vi "Main Editor UI.vi"() -> ()   [LabVIEW 2014, in "Missing Plugin editor node.lvclass"]
doc: "This is the main view for configuration the behavior of a module in the DCAF standard editor."
uses:
  Missing Plugin editor node.lvclass
  <vilib>/NI/Configuration Framework/Node/NodeRef.ctl
  <vilib>/NI/Configuration Framework/Node/NISE_CEF_Node.lvclass
  <vilib>/NI/AMC/Message Queue.ctl
  <vilib>/NI/AMC/Message.ctl
  <vilib>/NI/Tools/Keyed Array/KeyedArray.ctl
  <vilib>/NI/Configuration Framework/Node/UserEventRef.ctl
  <vilib>/NI/Configuration Framework/Controls/EventCluster.ctl
  <vilib>/NI/Configuration Framework/Node/StopEvent.ctl
  <vilib>/NI/Configuration Framework/Node/RefreshUIEvent.ctl
  <vilib>/NI/Configuration Framework/Node/CacheState.ctl
  <vilib>/NI/Configuration Framework/Node/NodeChangeEvent.ctl
  <vilib>/NI/DCAF/Tag Editor Core/Table API/Available Tag Menu/channel action event.ctl
  <vilib>/NI/DCAF/Tag Editor Core/Table API/Available Tag Menu/dialog output action.ctl
  <vilib>/NI/Tag Bus Module Framework/channel/TBM channel.lvclass
  <vilib>/NI/Tag Bus/tag/tag descriptor.lvclass
  <vilib>/NI/DCAF/Tag Editor Core/Table API/Table Manager/Call Back Ref Type Def.ctl
  <vilib>/NI/DCAF/Tag Editor Core/Configuration Editor/Classes/Engine Parent/Engine Parent Editor Node.lvclass
  <vilib>/NI/DCAF/Tag Editor Core/Configuration Editor/Classes/Module editor node/module editor node.lvclass
  <vilib>/NI/DCAF/Tag Editor Core/Table API/Table Manager/references.ctl
  module/configuration/Missing Plugin configuration.lvclass
  <vilib>/NI/Configuration Framework/serializable configuration/NISE_CEF_serializable configuration.lvclass
  <vilib>/NI/Configuration Framework/NISE_CEF_TreeControl.lvlib
  <vilib>/NI/Tools/Keyed Array/Tools_KeyedArray.lvlib
  <vilib>/NI/AMC/AMC.lvlib
  <vilib>/NI/DCAF/Tag Editor Core/Table API/Table Manager.lvlib
  <vilib>/NI/DCAF/Tag Editor Core/Table API/Table Manager/Table Manager.lvclass
  <vilib>/NI/DCAF UI Toolkit/Controls/DCAF UI Elements.lvlib
panel:
  out "Data":string
  in  "user event out":refnum<user-event>
  in  "node change":T1
  in  "cache state":T2
  in  "refresh UI":T3
  in  "stop event":T4
  in  "user event":T5
  in  "main queue":T6
  in  "node ref":T7
  # "Unable To Load Module"
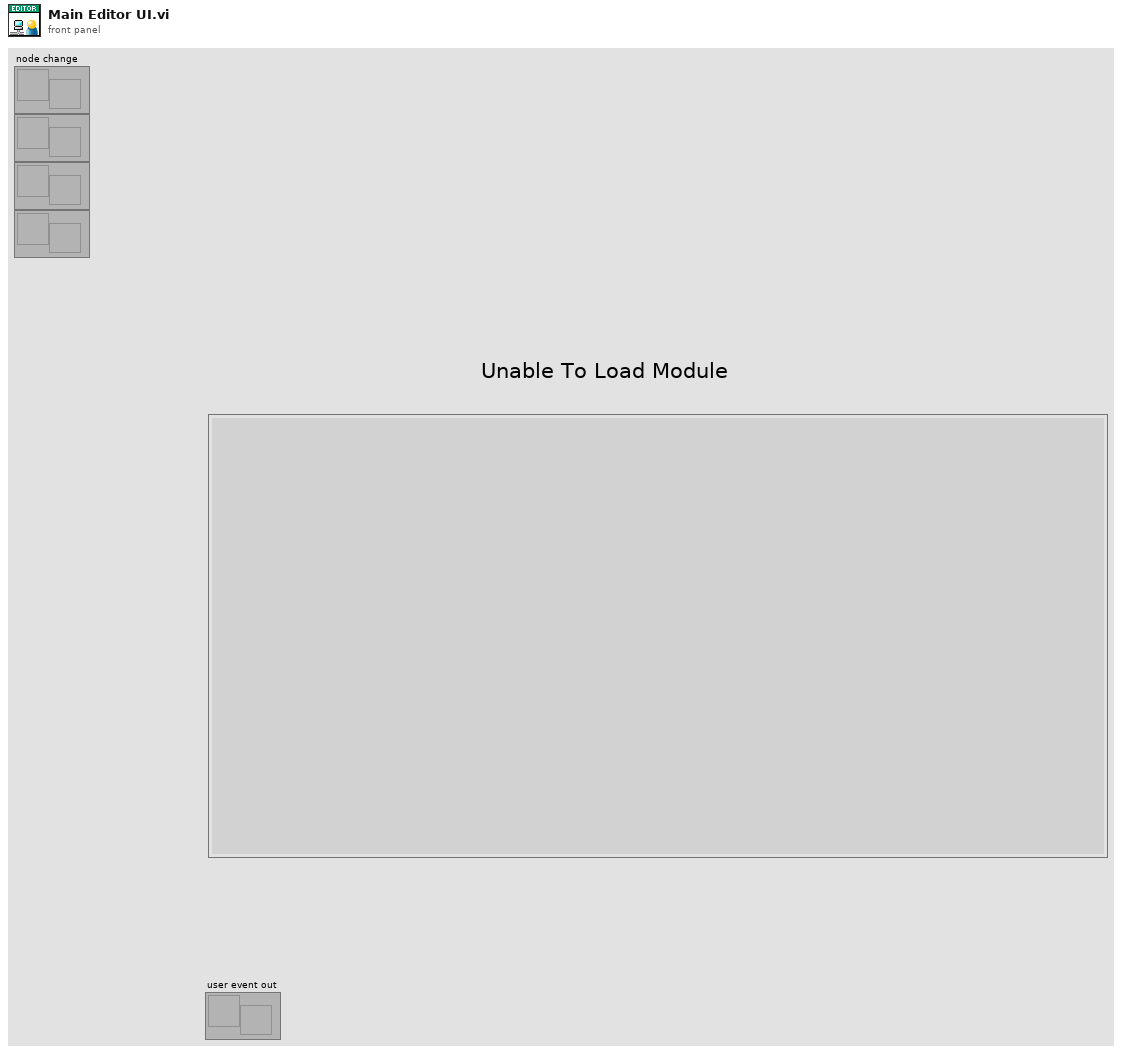
[diagram p1: front panel]
types:
  T1 = typedef "NISE_CEF_Node.lvclass/NodeChangeEvent.ctl" = refnum<user-event>
  T2 = typedef "NISE_CEF_Node.lvclass/CacheState.ctl" = refnum<user-event>
  T3 = typedef "NISE_CEF_Node.lvclass/RefreshUIEvent.ctl" = refnum<user-event>
  T4 = typedef "NISE_CEF_Node.lvclass/StopEvent.ctl" = refnum<user-event>
  T5 = typedef "NISE_CEF_Node.lvclass/UserEventRef.ctl" = refnum<user-event>
  T6 = typedef "AMC.lvlib/Message Queue.ctl" = refnum<queue>
  T7 = typedef "NISE_CEF_Node.lvclass/NodeRef.ctl" = refnum<data-value>
  T8 = typedef "Table Manager.lvlib/Table Manager.lvclass/references.ctl" = cluster{"stop event":T4, "refresh UI":T3, "cache state":T2, "node change":T1, "user event out":refnum<user-event>, "main queue":T6, "user event":T5}
  T9 = typedef "Table Manager.lvlib/Table Manager.lvclass/object ref.ctl" = cluster{"engine":refnum<data-value>, "Node Ref":refnum<data-value>}
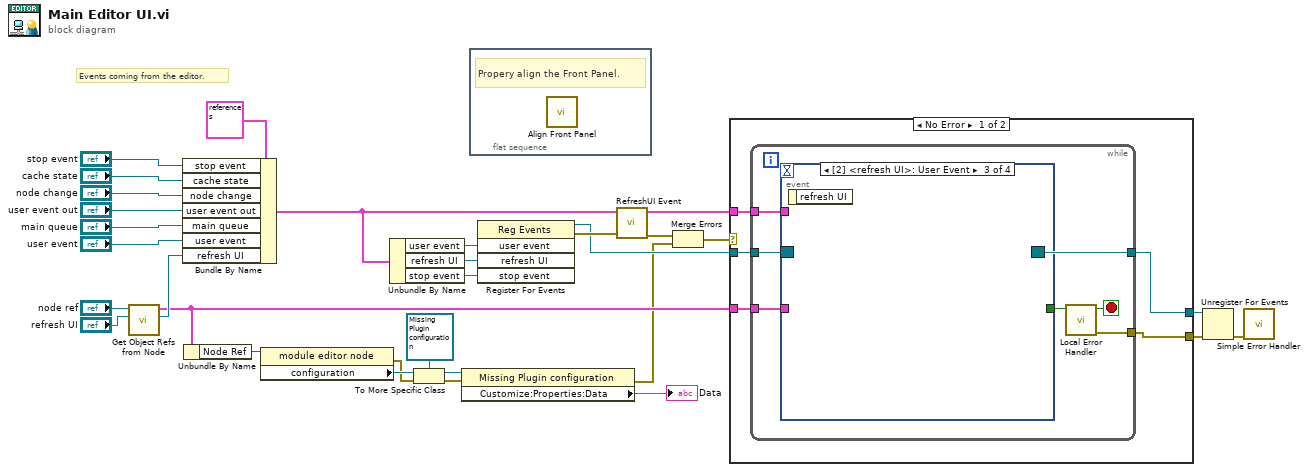
[diagram p0: block diagram]
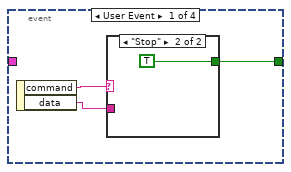
[diagram p2: hidden frame]
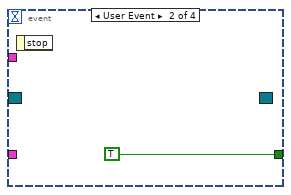
[diagram p4: hidden frame]
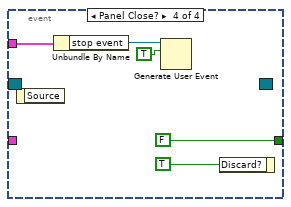
[diagram p5: hidden frame]
diagram:
  # "Events coming from the editor."
  n1 = call "Get Object Refs from Node.vi"("Refresh UI"="refresh UI", "Data Value Reference in"="node ref") -> ("Refresh UI out"=w17:T3, "References"=w10:T9)  [unwired: 7 in, 1 out]
  n2 = Bundle By Name(cluster=T8 {"stop event"=refnum, "refresh UI"=refnum, "cache state"=refnum, "node change"=refnum, "user event out"=refnum, "main queue"=refnum, "user event"=refnum} ("References"), "stop event"="stop event", "cache state"="cache state", "node change"="node change", "user event out"="user event out", "main queue"="main queue", "user event"="user event", "refresh UI"=w17) -> (w13:T8)
  n3 = Unbundle By Name(w10) -> ("Node Ref"=w9:refnum<data-value>)
  n4 = property class="module editor node"(reference=w9) -> (error out=w5:errorcluster, "configuration"=w8:refnum<class "NISE_CEF_serializable configuration.lvclass">)  [unwired: 1 in, 1 out]
  n5 = Unbundle By Name(w13) -> ("user event"=w16:T5, "refresh UI"=w15:T3, "stop event"=w14:T4)
  n6 = To More Specific Class(target class=refnum<class "Missing Plugin configuration.lvclass"> refnum ("Missing Plugin configuration"), reference=w8, error in=w5) -> (specific class reference=w6:refnum<class "Missing Plugin configuration.lvclass">, error out=w4:errorcluster)
  n7 = property class="Missing Plugin configuration"(reference=w6, error in=w4) -> (error out=w2:errorcluster, "Customize:Properties:Data"=→"Data":string)  [unwired: 1 out]
  n8 = flat-sequence {
    frame #0 {
      # "Propery align the Front Panel."
      n9 = call <vilib>:"Align Front Panel.vi"() -> ()  [unwired: 10 in, 2 out]
    }
  }
  n10 = register-events(w16, w15, w14) -> (reference out=w11:refnum<event-registration>, error out=w12:errorcluster)  [unwired: 2 in]
  n11 = call "RefreshUI Event.vi"("error in (no error)"=w12, "References in"=w13) -> ("error out"=w19:errorcluster, "References out"=w21:T8)  [unwired: 8 in]
  n12 = Merge Errors(w19, w2) -> (w3:errorcluster)
  n13 = case shown="No Error" w3 {
    selector: w3 -> [_ w55]
    tunnel: w11 -> [w36 w54]
    tunnel: [w35 w54] -> w31
    tunnel: [w32 w55] -> w30
    tunnel: w21 -> [w34 _]
    tunnel: w10 -> [w33 _]
    frame No Error {
      n14 = while {
        tunnel: w36 -> [w43]
        tunnel: [w42] -> w35
        tunnel: [w39] -> w32
        tunnel: w34 -> [w38]
        tunnel: w33 -> [w37]
        stop <- w41 stop-if-true
        n15 = event shown="[2] <refresh UI>: User Event" {
          selector: w43 -> [_ _ _ _]
          dyn-events: [_ _ _ _] -> w42
          timeout: _ -> [_ _ _ _]
          tunnel: [w46 TRUE _ FALSE] -> w40
          tunnel: w38 -> [_ _ _ w50]
          tunnel: w37 -> [_ _ _ _]
          event User Event {
            n16 = event-data() -> ("command"=w45:string, "data"=w44:string)  [unwired: 1 in]
            n17 = case shown="\"Stop\"" w45 {
              tunnel: [_ TRUE] -> w46
              tunnel: w44 -> [_ _]
              frame Default {
              }
              frame "Stop" {
              }
            }
          }
          event User Event {
            n18 = event-data() -> ()  [unwired: 1 in, 1 out]
          }
          event User Event {
            n19 = event-data() -> ()  [unwired: 1 in, 1 out]
          }
          event Panel Close? {
            n20 = event-data() -> ()  [unwired: 1 in, 1 out]
            n21 = Unbundle By Name(w50) -> ("stop event"=w49:T4)
            n22 = Generate User Event(user event=w49, event data cluster=TRUE ("event data")) -> ()  [unwired: 2 in, 2 out]
            n23 = event-data("Discard?"=TRUE) -> ()  [unwired: 1 in, 1 out]
          }
        }
        n24 = call "Local Error Handler.vi"("Stop in"=w40) -> ("error out"=w39:errorcluster, "Stop out"=w41:bool)  [unwired: 9 in]
      }
    }
    frame Error {
    }
  }
  n25 = Unregister For Events(event registration refnum=w31, error in=w30) -> (error out=w29:errorcluster)
  n26 = call <vilib>:"Simple Error Handler.vi"("error in (no error)"=w29) -> ()  [unwired: 4 in, 5 out]
